vi "PaneRelief.vi"   [LabVIEW 2015]
types:
  T1 = enum32{"Invalid", "Standard", "Closed", "Hidden", "Minimized", "Maximized"}
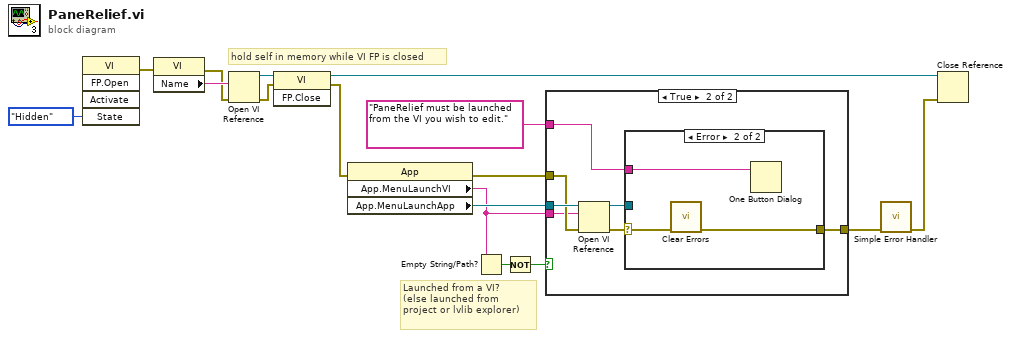
[diagram p0: block diagram]
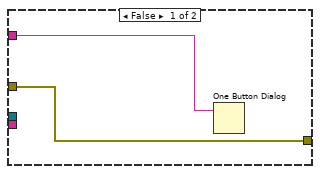
[diagram p2: hidden frame]
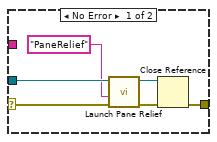
[diagram p3: hidden frame]
diagram:
  # "hold self in memory while VI FP is closed"
  # "Launched from a VI?\n(else launched from project or lvlib explorer)"
  n1 = invoke class="VI" method="FP.Open"("State"=T1."Hidden") -> (error out=w2:errorcluster)  [unwired: 4 in, 4 out]
  n2 = property class="VI"(error in=w2) -> (error out=w3:errorcluster, "Name"=w9:string)  [unwired: 1 in, 1 out]
  n3 = Open VI Reference(vi path=w9, error in (no error)=w3) -> (vi reference=w8:refnum<vi>, error out=w5:errorcluster)  [unwired: 4 in]
  n4 = invoke class="VI" method="FP.Close"(reference=w8, error in=w5) -> (reference out=w6:refnum<vi>, error out=w10:errorcluster)  [unwired: 1 in, 1 out]
  n5 = property class="App"(error in=w10) -> (error out=w15:errorcluster, "App.MenuLaunchVI"=w14:string, "App.MenuLaunchApp"=w16:refnum<vi>)  [unwired: 1 in, 1 out]
  n6 = Empty String/Path?(string/path=w14) -> (empty?=w13:bool)
  n7 = Not(x=w13) -> (.not. x?=w12:bool)
  n8 = case shown="True" w12 {
    tunnel: w16 -> [_ w25]
    tunnel: w15 -> [w18 w23]
    tunnel: w14 -> [_ w21]
    tunnel: [w18 w20] -> w11
    tunnel: "PaneRelief must be launched from the VI you wish to edit." ("message") -> [w17 w19]
    frame False {
      n9 = One Button Dialog(message=w17) -> ()  [unwired: 1 in, 1 out]
    }
    frame True {
      n10 = Open VI Reference(application reference (local)=w25, vi path=w21, error in (no error)=w23) -> (vi reference=w24:refnum<vi>, error out=w22:errorcluster)  [unwired: 3 in]
      n11 = case shown="Error" w22 {
        selector: w22 -> [w28 w34]
        tunnel: w24 -> [w31 _]
        tunnel: [w27 w33] -> w20
        tunnel: w19 -> [_ w32]
        frame No Error {
          n12 = call "Launch Pane Relief.vi"("error in (no error)"=w28, "Undo Transaction Name"="PaneRelief", "VI in"=w31) -> ("error out"=w29:errorcluster, "VI out"=w30:refnum<vi>)  [unwired: 7 in]
          n13 = Close Reference(reference=w30, error in (no error)=w29) -> (error out=w27:errorcluster)
        }
        frame Error {
          n14 = call <vilib>:"Clear Errors.vi"("error in (no error)"=w34) -> ("error out"=w33:errorcluster)  [unwired: 5 in, 1 out]
          n15 = One Button Dialog(message=w32) -> ()  [unwired: 1 in, 1 out]
        }
      }
    }
  }
  n16 = call <vilib>:"Simple Error Handler.vi"("error in (no error)"=w11) -> ("error out"=w7:errorcluster)  [unwired: 4 in, 4 out]
  n17 = Close Reference(reference=w6, error in (no error)=w7) -> ()  [unwired: 1 out]
